vi "Locate in Project.vi"(6 "Mouse Position":T1 caption="鼠标位置", 7 "User VI Ref":refnum<vi> caption="用户VI引用", 8 "Is Multi-select?":bool caption="为多选？", 9 "Remaining Items":refnum<vi>[](array[refnum]) caption="剩余项", 10 "Affected Items":T8 caption="受影响的项", 11 "Menu Refnum":refnum<k9> caption="菜单引用句柄") -> (3 "Menu Items To Add":T2[](array[typedef]) caption="待添加菜单项")   [LabVIEW 2020]
doc: "该VI属于修改LabVIEW快捷菜单部分。这是创建快捷菜单时调用的生成VI。该VI为LabVIEW输入添加到菜单的快捷菜单项。"
uses:
  <resource>/plugins/PopupMenus/support/Shortcut Menu Item Definition.ctl
  <resource>/plugins/PopupMenus/support/Transaction Control.ctl
  <resource>/plugins/PopupMenus/support/Position In Menu.ctl
  <resource>/plugins/PopupMenus/support/Relative Position.ctl
  <resource>/plugins/PopupMenus/support/Checkmark Status.ctl
  <resource>/plugins/PopupMenus/support/Enabled Menu Item Status.ctl
  Locate in Project.ctl
  <vilib>/Utility/miscctls.llb/LVPositionTypeDef.ctl
panel:
  # "弹出插件时必须遵循的规则：\n*该VI的文件名称必须与LLB的文件名称匹配－不同的只是文件扩展名。\n*VI必须禁用调试，否则它将作为插件被忽略。\n*所有菜单项的“标签后缀 + VI文件名”必须少于240个字符。\n*可从自定义类型断开连接“受影响的项”，从而加快插件的加载速度。存在该自定义类型的目的是使该VI和执行VI使用相同的类型。\n*除“受影响的项”之外，前面板上的其他所有控件都已锁定，以防被意外编辑。除“受影响的项”簇中的元素外，不要修改控件的类型或名称。\n*请参考即时帮助，了解每个控件的详细信息。"
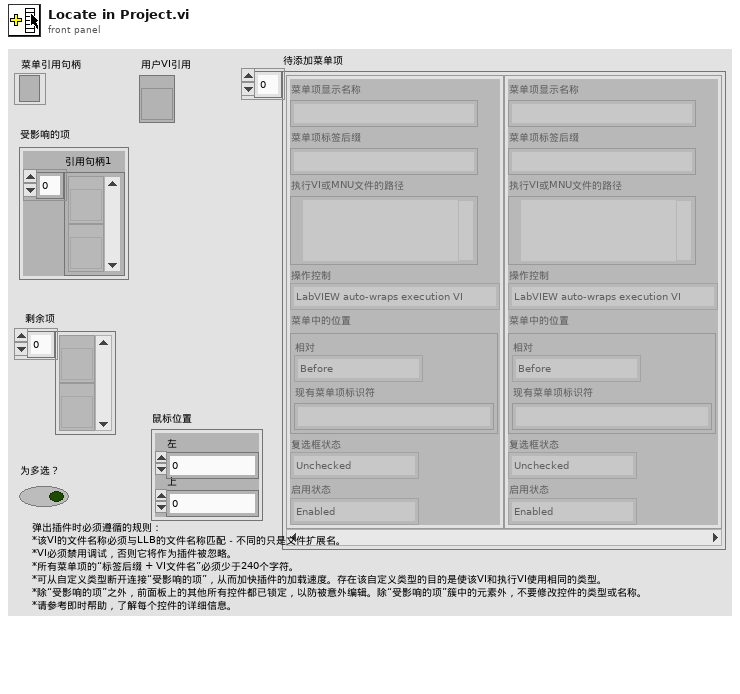
[diagram p1: front panel]
types:
  T1 = typedef "LVPositionTypeDef.ctl" = cluster{"Left":i32, "Top":i32}
  T2 = typedef "Shortcut Menu Item Definition.ctl" = cluster{"Menu Item Display Name":string, "Menu Item Tag Suffix":string, "Path To Execution VI or MNU":path, "Transaction Control":T3, "Position In Menu":T4, "Checkmark Status":T6, "Enabled Status":T7}
  T3 = typedef "Transaction Control.ctl" = enum8{"LabVIEW auto-wraps execution VI", "Execution VI will define if needed"}
  T4 = typedef "Position In Menu.ctl" = cluster{"Relative":T5, "Existing Item Tag":string}
  T5 = typedef "Relative Position.ctl" = enum8{"Before", "Instead of", "After", "Into Submenu"}
  T6 = typedef "Checkmark Status.ctl" = enum8{"Unchecked", "Checked"}
  T7 = typedef "Enabled Menu Item Status.ctl" = enum8{"Enabled", "Disabled"}
  T8 = typedef "Locate in Project.ctl" = cluster{"Refnums 1":refnum<vi>[]}
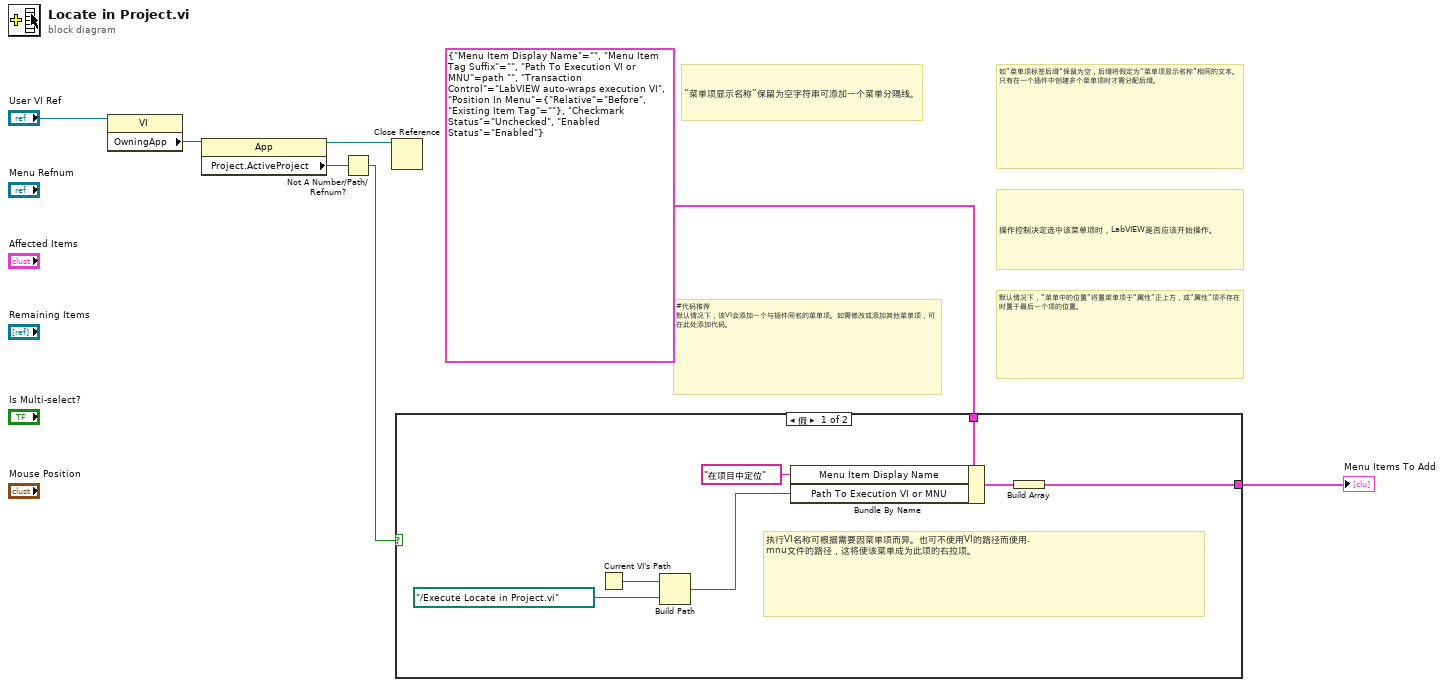
[diagram p0: block diagram]
diagram:
  # "操作控制决定选中该菜单项时，LabVIEW是否应该开始操作。"
  # "#代码推荐 默认情况下，该VI会添加一个与插件同名的菜单项。如需修改或添加其他菜单项，可在此处添加代码。"
  # "“菜单项显示名称”保留为空字符串可添加一个菜单分隔线。"
  # "如”菜单项标签后缀“保留为空，后缀将假定为“菜单项显示名称”相同的文本。只有在一个插件中创建多个菜单项时才需分配后缀。"
  # "默认情况下，“菜单中的位置”将置菜单项于“属性”正上方，或“属性”项不存在时置于最后一个项的位置。"
  n1 = property class="VI"(reference="User VI Ref") -> ("OwningApp"=w4:refnum<vi>)  [unwired: 1 in, 2 out]
  n2 = property class="App"(reference=w4) -> (reference out=w1:refnum<vi>, "Project.ActiveProject"=w3:refnum<vi>)  [unwired: 1 in, 1 out]
  n3 = Not A Number/Path/Refnum?(number/path/refnum=w3) -> (NaN/Path/Refnum?=w2:bool)
  n4 = Close Reference(reference=w1) -> ()  [unwired: 1 in, 1 out]
  n5 = case shown="假" w2 {
    tunnel: T2 {"Menu Item Display Name"="", "Menu Item Tag Suffix"="", "Path To Execution VI or MNU"=path "", "Transaction Control"=enum."LabVIEW auto-wraps execution VI", "Position In Menu"={"Relative"=enum."Before", "Existing Item Tag"=""}, "Checkmark Status"=enum."Unchecked", "Enabled Status"=enum."Enabled"} ("Cluster") -> [w12 _]
    tunnel: [w10 _] -> w6
    frame False {
      # "执行VI名称可根据需要因菜单项而异。也可不使用VI的路径而使用.mnu文件的路径，这将使该菜单成为此项的右拉项。"
      n6 = Current VI's Path() -> (path=w9:path)
      n7 = Build Path(base path=w9, name or relative path=path "../Execute Locate in Project.vi" ("execute path")) -> (appended path=w13:path)
      n8 = Bundle By Name(cluster=w12, "Menu Item Display Name"="在项目中定位", "Path To Execution VI or MNU"=w13) -> (w11:T2)
      n9 = Build Array(w11) -> (w10:T2[])
    }
    frame True {
    }
  }
  "Menu Items To Add" <- w6
